vi "Extensions to Browse Pattern.vi"(11 "extensions":string[](array[string])) -> (3 "spreadsheet string":string)   [LabVIEW 2011, in "Engine Sim System Explorer.lvlib"]
uses:
  Engine Sim System Explorer.lvlib
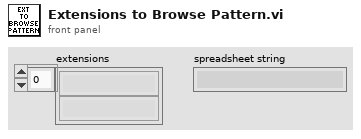
[diagram p1: front panel]
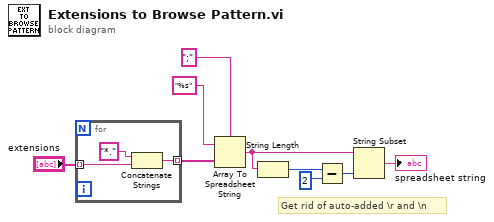
[diagram p0: block diagram]
diagram:
  # "Get rid of auto-added \\r and \\n"
  n1 = for {
    tunnel: "extensions" -> [w12] mode=indexing
    tunnel: [w10] -> w6 mode=indexing
    n2 = Concatenate Strings("*." ("string"), w12) -> (w10:string)
  }
  n3 = Array To Spreadsheet String(delimiter (Tab)=";", array=w6, 3:"%s" ("format string")) -> (spreadsheet string=w4:string)
  n4 = String Length(string=w4) -> (length=w3:i32)
  n5 = Subtract(x=w3, y=2) -> (x-y=w1:i32)
  n6 = String Subset(string=w4, length (rest)=w1) -> (substring=→"spreadsheet string":string)  [unwired: 1 in]
